vi "Input Impedence_Freq Domian(SubVI).vi"(7 "Settings":T1={"Min. Hrmonic for Zc"=4.0, "Max. Harmonic for Zc"=10.0}, 10 "Flow Rate (ml/s)":waveform(dbl), 11 "Pressure (mmHg)":waveform(dbl)) -> (0 "Zo (at 0 Hz) (mmHg/ml/s)":dbl, 1 "Zc (mmHg/ml/s)":dbl format="%0.2f", 2 "Zo - Phase Spectrum":waveform(dbl)(graph)={"t0"=timestamp(0 s since 1904-01-01), "dt"=1.2484394506866416, "Y"=array[801 elements]}, 3 "Zo - Magnitude Spectrum":waveform(dbl)(graph)={"t0"=timestamp(0 s since 1904-01-01), "dt"=1.2484394506866416, "Y"=array[801 elements]})   [LabVIEW 2017]
uses:
  <vilib>/Analysis/NI_AALPro.lvlib
  <vilib>/Analysis/2dsp.llb/Real FFT.vi
  <vilib>/Analysis/NI_AALBase.lvlib
  <vilib>/Analysis/baseanly.llb/Mean (DBL).vi
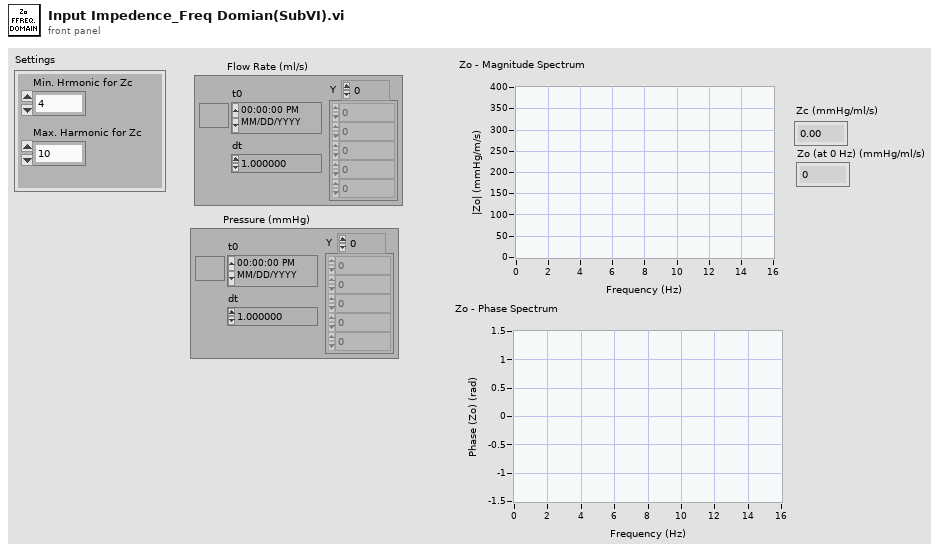
[diagram p1: front panel]
types:
  T1 = cluster{"Min. Hrmonic for Zc":dbl, "Max. Harmonic for Zc":dbl}
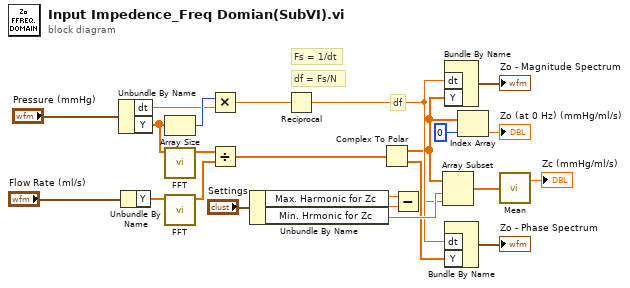
[diagram p0: block diagram]
diagram:
  # "Fs = 1/dt"
  # "df = Fs/N"
  # "df"
  n1 = Unbundle By Name("Pressure (mmHg)") -> ("dt"=w9:dbl, "Y"=w11:dbl[])
  n2 = Unbundle By Name("Flow Rate (ml/s)") -> ("Y"=w12:dbl[])
  n3 = Array Size(array=w11) -> (size(s)=w10:i32)
  n4 = call-poly <vilib>:"FFT.vi"("X"=w11) -> ("FFT {X}"=w18:cdb[])  [unwired: 9 in, 1 out]
  n5 = call-poly <vilib>:"FFT.vi"("X"=w12) -> ("FFT {X}"=w17:cdb[])  [unwired: 9 in, 1 out]
  n6 = Multiply(x=w10, y=w9) -> (x*y=w8:dbl)
  n7 = Divide(x=w18, y=w17) -> (x/y=w16:cdb[])
  n8 = Unbundle By Name("Settings") -> ("Max. Harmonic for Zc"=w19:dbl, "Min. Hrmonic for Zc"=w20:dbl)
  n9 = Reciprocal(x=w8) -> (1/x=w7:dbl)
  n10 = Complex To Polar(r * e^(i*theta)=w16) -> (r=w3:dbl[], theta=w15:dbl[])
  n11 = Subtract(x=w19, y=w20) -> (x-y=w6:dbl)
  n12 = Array Subset(array=w3, index=w20, length=w6) -> (w5:dbl[])
  n13 = Bundle By Name("dt"=w7, "Y"=w3) -> (→"Zo - Magnitude Spectrum":waveform(dbl))  [unwired: 1 in]
  n14 = Bundle By Name("dt"=w7, "Y"=w15) -> (→"Zo - Phase Spectrum":waveform(dbl))  [unwired: 1 in]
  n15 = Index Array(array=w3, index=0) -> (element=→"Zo (at 0 Hz) (mmHg/ml/s)":dbl)
  n16 = call-poly <vilib>:"Mean.vi"("X"=w5) -> ("mean"=→"Zc (mmHg/ml/s)":dbl)  [unwired: 1 out]
